vi "Create Queue.vi"(9 "Queue jettl":refnum<class "Queue jettl.lvclass">, 10 "Alias":string, 11 "Base Queue jettl in":refnum<class "Base Queue jettl.lvclass">) -> (3 "Base Queue jettl out":refnum<class "Base Queue jettl.lvclass">)   [LabVIEW 2021, in "jettl.lvlib" / "Base Queue jettl.lvlib" / "Base Queue jettl.lvclass"]
uses:
  Base Queue jettl.lvclass
  Queue jettl/Queue jettl.lvclass
  Msg Strategy/Msg Strategy.lvclass
  Base Queue jettl.lvclass/Base Queue jettl.ctl
  jettl.lvlib
  Queue Mailbox/Queue Mailbox.lvlib
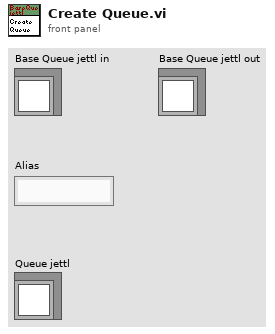
[diagram p1: front panel]
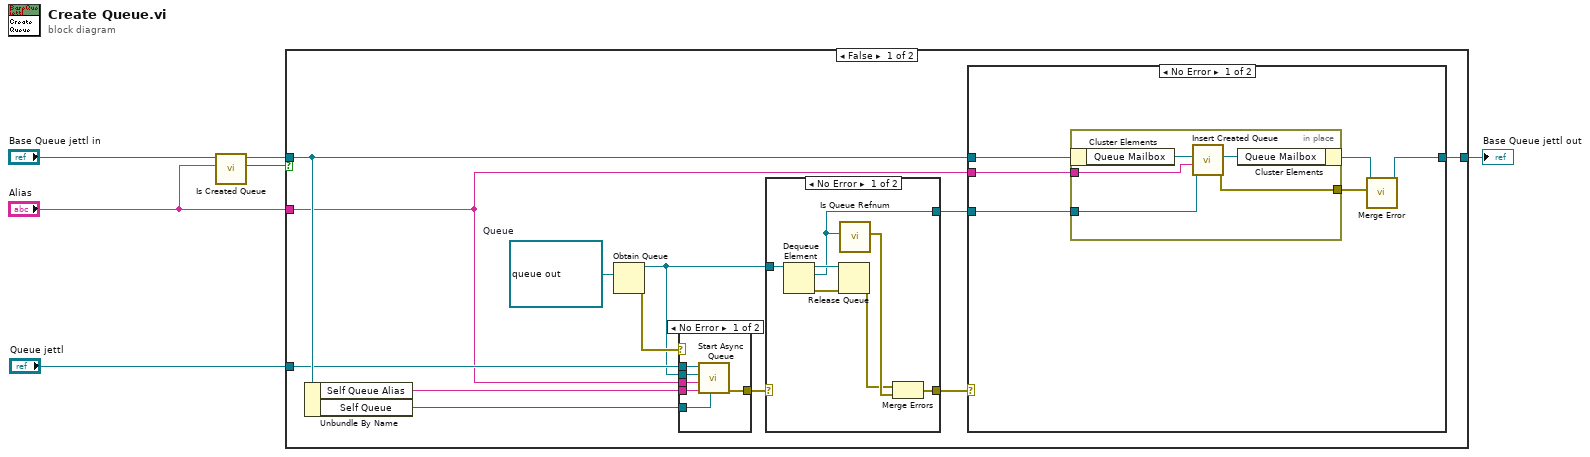
[diagram p0: block diagram]
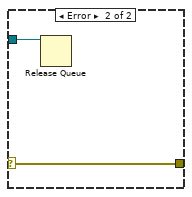
[diagram p2: hidden frame]
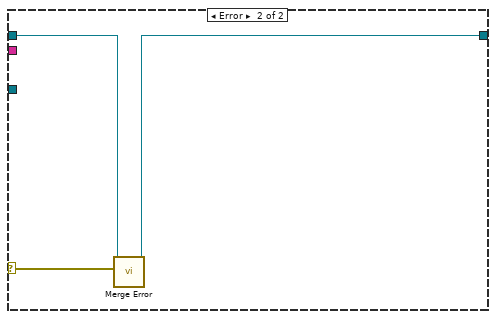
[diagram p4: hidden frame]
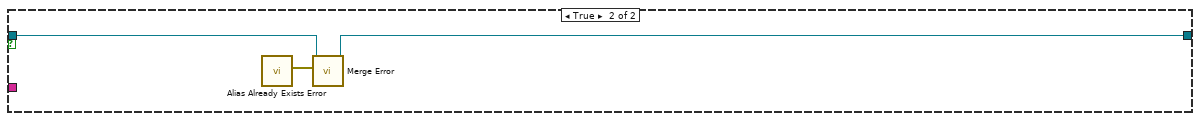
[diagram p5: hidden frame]
diagram:
  n1 = call-dynamic "Is Created Queue.vi"("Created Queue Alias"="Alias", "Base Queue jettl in"="Base Queue jettl in") -> ("Is Created Queue?"=w4:bool, "Base Queue jettl out"=w3:refnum<class "Base Queue jettl.lvclass">)  [unwired: 8 in]
  n2 = case shown="False" w4 {
    tunnel: "Queue jettl" -> [w16 _]
    tunnel: w3 -> [w18 w51]
    tunnel: "Alias" -> [w15 _]
    tunnel: [w17 w50] -> w6
    frame False {
      w9 = refnum<data-value> refnum  # Queue
      n3 = Unbundle By Name(w18) -> ("Self Queue Alias"=w8:string, "Self Queue"=w7:refnum<data-value>)
      n4 = Obtain Queue(element data type=w9) -> (queue out=w11:refnum<queue>, error out=w14:errorcluster)  [unwired: 4 in, 1 out]
      n5 = case shown="No Error" w14 {
        selector: w14 -> [_ w34]
        tunnel: [w32 w34] -> w12
        tunnel: w16 -> [w33 _]
        tunnel: w11 -> [w31 _]
        tunnel: w15 -> [w30 _]
        tunnel: w8 -> [w29 _]
        tunnel: w7 -> [w28 _]
        frame No Error {
          n6 = call "Start Async Queue.vi"("Creator"=w28, "Creator Alias"=w29, "Self Alias"=w30, "Queue of Queue Self"=w31, "Queue jettl"=w33) -> ("error out"=w32:errorcluster)  [unwired: 6 in]
        }
        frame Error {
        }
      }
      n7 = case shown="No Error" w12 {
        selector: w12 -> [_ w27]
        tunnel: [w23 w27] -> w13
        tunnel: w11 -> [w20 w26]
        tunnel: [w19 _] -> w10
        frame No Error {
          n8 = Dequeue Element(queue=w20) -> (queue out=w24:refnum<queue>, element=w19:refnum<data-value>, error out=w25:errorcluster)  [unwired: 2 in, 1 out]
          n9 = Release Queue(queue=w24, error in (no error)=w25) -> (error out=w21:errorcluster)  [unwired: 1 in, 2 out]
          n10 = call "Is Queue Refnum.vi"("Queue"=w19) -> ("Error"=w22:errorcluster)  [unwired: 10 in]
          n11 = Merge Errors(w21, w22) -> (w23:errorcluster)
        }
        frame Error {
          n12 = Release Queue(queue=w26) -> ()  [unwired: 2 in, 3 out]
        }
      }
      n13 = case shown="No Error" w13 {
        selector: w13 -> [_ w46]
        tunnel: w18 -> [w37 w48]
        tunnel: [w38 w47] -> w17
        tunnel: w10 -> [w40 _]
        tunnel: w15 -> [w39 _]
        frame No Error {
          n14 = in-place {
            in-place-border: w40 -> [w42]
            in-place-border: w39 -> [w43]
            in-place-border: [w41] -> w35
            n15 = in-place-cluster #1(w37) -> ("Queue Mailbox"=w45:refnum<data-value>)
            n16 = call "Insert Created Queue.vi"("Self Queue"=w42, "Self Queue Alias"=w43, "Queue Mailbox in"=w45) -> ("error out"=w41:errorcluster, "Queue Mailbox out"=w44:refnum<data-value>)  [unwired: 7 in]
            n17 = in-place-cluster #1("Queue Mailbox"=w44) -> (w36:refnum<class "Base Queue jettl.lvclass">)
          }
          n18 = call-dynamic "Merge Error.vi"("Error"=w35, "Base Queue jettl in"=w36) -> ("Base Queue jettl out"=w38:refnum<class "Base Queue jettl.lvclass">)  [unwired: 9 in]
        }
        frame Error {
          n19 = call-dynamic "Merge Error.vi"("Error"=w46, "Base Queue jettl in"=w48) -> ("Base Queue jettl out"=w47:refnum<class "Base Queue jettl.lvclass">)  [unwired: 9 in]
        }
      }
    }
    frame True {
      n20 = call "Alias Already Exists Error.vi"() -> ("Error"=w49:errorcluster)  [unwired: 11 in]
      n21 = call-dynamic "Merge Error.vi"("Error"=w49, "Base Queue jettl in"=w51) -> ("Base Queue jettl out"=w50:refnum<class "Base Queue jettl.lvclass">)  [unwired: 9 in]
    }
  }
  "Base Queue jettl out" <- w6
